vi "Open Document.vi"(8 "error in (no error)":errorcluster, 10 "File Path":path, 11 "Document in":refnum<class "Document.lvclass">) -> (0 "error out":errorcluster, 3 "Document out":refnum<class "Document.lvclass">)   [LabVIEW 2020, in "LabVIEW NPOI.lvlib" / "Document.lvclass"]
doc: "Opens the <b>Document</b> file located at <b>File Path</b> for reading.\n\nNotes:\n - If <b>File Path</b> is empty (default) or is <Not A Path> or is a directory, error 7 is returned."
uses:
  Document.lvclass
  Document.lvclass/Document.ctl
  Set FilePath.vi
  <vilib>/Utility/error.llb/Error Cluster From Error Code.vi
  <vilib>/ErrorRing/Error Ring.xnode
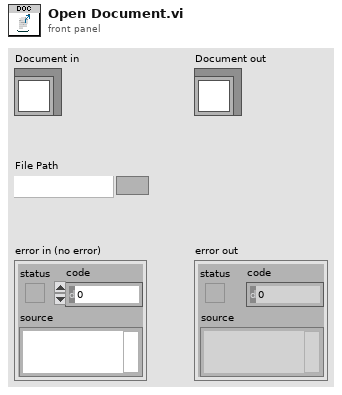
[diagram p1: front panel]
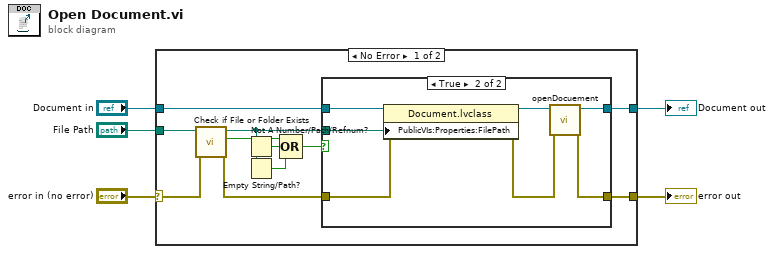
[diagram p0: block diagram]
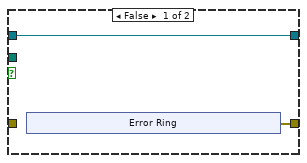
[diagram p2: hidden frame]
diagram:
  n1 = case shown="No Error" "error in (no error)" {
    selector: "error in (no error)" -> [w12 w31]
    tunnel: [w14 w31] -> w4
    tunnel: [w15 w30] -> w2
    tunnel: "Document in" -> [w16 w30]
    tunnel: "File Path" -> [w13 _]
    frame No Error {
      n2 = call <vilib>:"Check if File or Folder Exists.vi"("error in (no error)"=w12, "path"=w13) -> ("error out"=w11:errorcluster, "file or folder exists?"=w7:bool, "dup path"=w8:path)  [unwired: 7 in]
      n3 = Not A Number/Path/Refnum?(number/path/refnum=w8) -> (NaN/Path/Refnum?=w10:bool)
      n4 = Empty String/Path?(string/path=w8) -> (empty?=w9:bool)
      n5 = Compound Arithmetic op=OR(w7, w10, w9) -> (w6:bool)
      n6 = case shown="True" w6 {
        tunnel: w16 -> [w18 w27]
        tunnel: [w18 w29] -> w15
        tunnel: [w17 w28] -> w14
        tunnel: w11 -> [_ w24]
        tunnel: w8 -> [_ w25]
        frame False {
          n7 = xnode "Error Ring"() -> ("error out"=w17:errorcluster)
        }
        frame True {
          n8 = property class="Document.lvclass"(reference=w27, error in=w24, "PublicVIs:Properties:FilePath"=w25) -> (reference out=w26:refnum<class "Document.lvclass">, error out=w23:errorcluster)
          n9 = call-dynamic "openDocuement.vi"("error in (no error)"=w23, "Document in"=w26) -> ("error out"=w28:errorcluster, "Document out"=w29:refnum<class "Document.lvclass">)  [unwired: 8 in]
        }
      }
    }
    frame Error {
    }
  }
  "error out" <- w4
  "Document out" <- w2
